vi "Tau(x).vi"(10 "X":dbl) -> (2 "Tau":dbl)   [LabVIEW 2014]
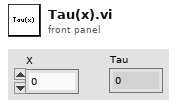
[diagram p1: front panel]
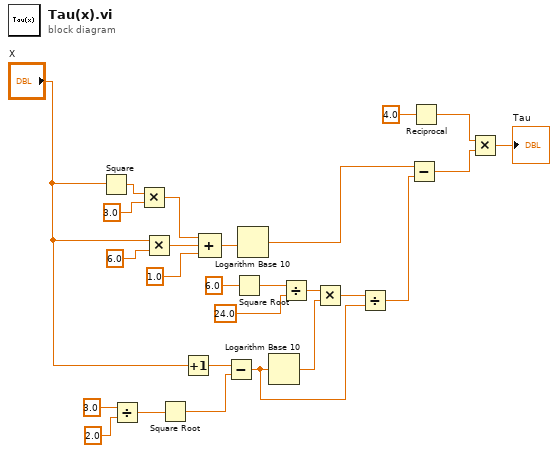
[diagram p0: block diagram]
diagram:
  n1 = Square(x="X") -> (x^2=w25:dbl)
  n2 = Divide(x=3.0, y=2.0) -> (x/y=w12:dbl)
  n3 = Multiply(x=w25, y=3.0) -> (x*y=w24:dbl)
  n4 = Multiply(x="X", y=6.0) -> (x*y=w22:dbl)
  n5 = Square Root(x=w12) -> (sqrt(x)=w13:dbl)
  n6 = Increment(x="X") -> (x+1=w14:dbl)
  n7 = Compound Arithmetic op=ADD(w24, w22, 1.0 ("value")) -> (w19:dbl)
  n8 = Subtract(x=w14, y=w13) -> (x-y=w5:dbl)
  n9 = Square Root(x=6.0) -> (sqrt(x)=w9:dbl)
  n10 = Logarithm Base 10(1:w19) -> (0:w18:dbl)
  n11 = Logarithm Base 10(1:w5) -> (0:w7:dbl)
  n12 = Divide(x=w9, y=24.0) -> (x/y=w16:dbl)
  n13 = Multiply(x=w16, y=w7) -> (x*y=w6:dbl)
  n14 = Divide(x=w6, y=w5) -> (x/y=w4:dbl)
  n15 = Subtract(x=w18, y=w4) -> (x-y=w2:dbl)
  n16 = Reciprocal(x=4.0) -> (1/x=w3:dbl)
  n17 = Multiply(x=w3, y=w2) -> (x*y=→"Tau":dbl)
